vi "Read VI and FP Refs.vi"(0 "GUI View in":refnum<class "GUI View.lvclass">, 7 "View Hierarchy Level":i32, 11 "error in (no error)":errorcluster) -> (4 "GUI View out":refnum<class "GUI View.lvclass">, 6 "VI Ref":refnum<vi>, 8 "FP Ref":refnum<vi>, 10 "View Found":bool, 15 "error out":errorcluster)   [LabVIEW 2023, in "GUI Views.lvlib" / "GUI View.lvclass"]
uses:
  GUI View.lvclass
  <userlib>/_OpenG.lib/error/error.llb/openg_error.lvlib
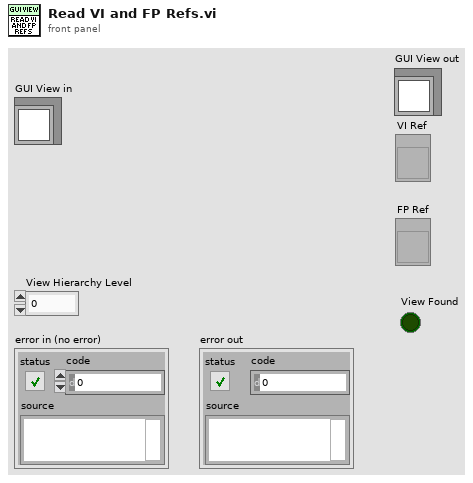
[diagram p1: front panel]
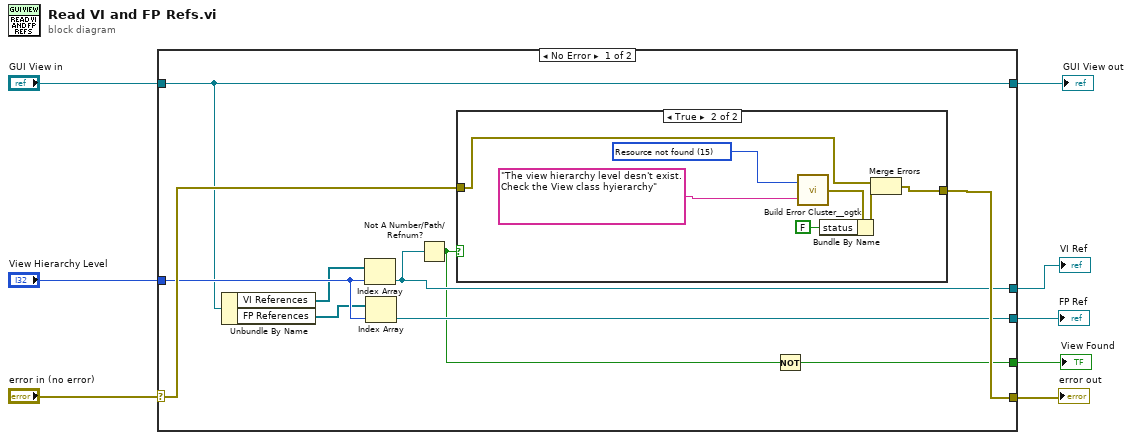
[diagram p0: block diagram]
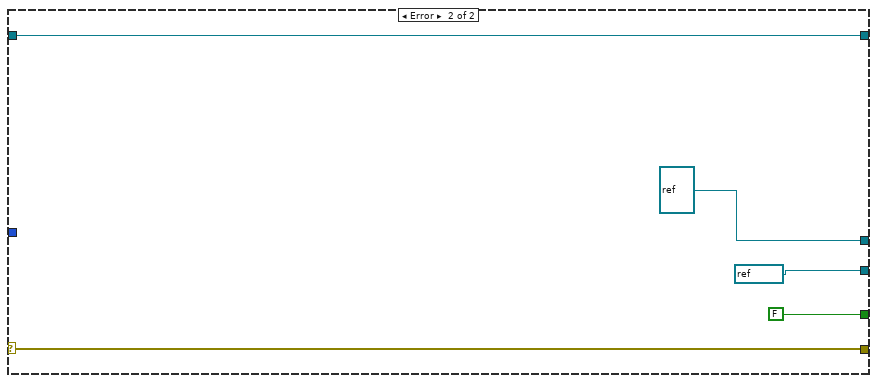
[diagram p3: hidden frame]
diagram:
  n1 = case shown="No Error" "error in (no error)" {
    selector: "error in (no error)" -> [w17 w30]
    tunnel: [w18 w30] -> w8
    tunnel: "GUI View in" -> [w10 w31]
    tunnel: "View Hierarchy Level" -> [w16 _]
    tunnel: [w10 w31] -> w4
    tunnel: [w15 refnum<vi> refnum ("Panel")] -> w3
    tunnel: [w14 refnum<vi> refnum ("reference out")] -> w2
    tunnel: [w9 FALSE] -> w1
    frame No Error {
      n2 = Unbundle By Name(w10) -> ("VI References"=w12:refnum<vi>[], "FP References"=w11:refnum<vi>[])
      n3 = Index Array(array=w12, index=w16) -> (element=w14:refnum<vi>)
      n4 = Index Array(array=w11, index=w16) -> (element=w15:refnum<vi>)
      n5 = Not A Number/Path/Refnum?(number/path/refnum=w14) -> (NaN/Path/Refnum?=w13:bool)
      n6 = case shown="True" w13 {
        tunnel: w17 -> [w19 w25]
        tunnel: [w19 w23] -> w18
        frame False {
        }
        frame True {
          w26 = 15 items=["No error", "Argument error", "Memory is full", "Out of zone", "End of file", "File already open", "Generic file I/O error", "File not found", "File permission error", "Disk is full", "Duplicate path", "Too many files open", "System feature not enabled", "Resource file not found", "Cannot add resource", "Resource not found", "Image not found", "Image memory error", "Pen does not exist", "Config type invalid", "Config token not found", "Config parse error", "Config memory error", "Bad external code format", "Bad external code offset", "External code not present", "Null window", "Destroy window error", "Null menu", "Print aborted", "Bad print record", "Print driver error", "Windows error during printing", "Memory error during printing", "Print dialog error", "Generic print error", "Invalid device refnum", "Device not found", "Device parameter error", "Device unit error", "Cannot open device", "Device call aborted", "Generic error", "Cancelled by user", "Object ID too low", "Object ID too high", "Object not in heap", "Unknown heap", "Unknown object (invalid DefProc)", "Unknown object (DefProc not in table)", "Message out of range", "Invalid (null) method", "Unknown message", "Manager call not supported", "Bad address", "Network operation in progress", "Network operation timed out", "Connection is busy", "Network attribute not supported", "Network error", "Address in use", "System out of memory", "Connection aborted", "Connection refused", "Not connected", "Already connected", "Connection closed", "Initialization error (interapplication manager)", "Bad occurrence", "Wait on unbound occurrence handler", "Occurrence queue overflow", "Datalog type conflict", "Unused", "Unrecognized type (interapplication manager)", "Memory corrupt", "Failed to make temporary DLL", "Old CIN version", "Drag socket not found", "Failed to load drop-object", "Failed to register OLE object", "Failed to release OLE object", "Format specifier type mismatch", "Unknown format specifier", "Too few format specifiers", "Too many format specifiers", "Scan failed", "Newer CIN version", "Error converting to variant", "Runtime menu error", "Password tampered", "Variant attribute not found", "Incompatible variant data type", "Event data is not available", "Event Store is not present", "Occurrence is not found", "Event Queue is not created", "Event info is not available", "Refnum passed is NULL", "Error retrieving Class GUID", "Error retrieving CoClass GUID", "Error retrieving TypeLib GUID.", "Bad built application magic bytes.", "Specific driver is different from the specific driver associated with the Logical Name.", "There is no session opened to the class driver.", "Max Error", "MAX - Error with config objects", "MAX - Error loading configuration", "MAX - Group not supported"]
          n7 = call <userlib>:"Build Error Cluster__ogtk.vi"("String to Prepend to source (\"\")"="The view hierarchy level desn't exist. Check the View class hyierarchy" ("String to Prepend to source (\"\")"), "code"=w26) -> ("error out"=w24:errorcluster)
          n8 = Bundle By Name(cluster=w24, "status"=FALSE) -> (w21:errorcluster)
          n9 = Merge Errors(w25, w21) -> (w23:errorcluster)
        }
      }
      n10 = Not(x=w13) -> (.not. x?=w9:bool)
    }
    frame Error {
    }
  }
  "error out" <- w8
  "GUI View out" <- w4
  "FP Ref" <- w3
  "VI Ref" <- w2
  "View Found" <- w1
